vi "Unquote.vi"(1 "String":string) -> (0 "trimmed string":string)   [LabVIEW 2023, in "LV ArgParse.lvlib" / "LV Argument Parser.lvclass"]
uses:
  LV Argument Parser.lvclass
  <vilib>/Utility/error.llb/Trim Whitespace One-Sided.vi
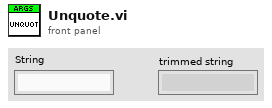
[diagram p1: front panel]
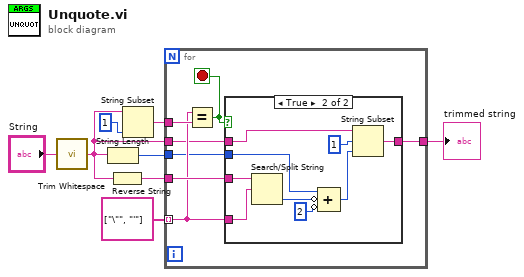
[diagram p0: block diagram]
diagram:
  n1 = call <vilib>:"Trim Whitespace.vi"("string"="String") -> ("trimmed string"=w2:string)  [unwired: 1 in]
  n2 = String Length(string=w2) -> (length=w3:i32)
  n3 = Reverse String(1:w2) -> (0:w5:string)
  n4 = String Subset(string=w2, length (rest)=1 ("length (rest)")) -> (substring=w6:string)  [unwired: 1 in]
  n5 = for {
    tunnel: w6 -> [w15]
    tunnel: w5 -> [w14]
    tunnel: string[] ["\"", "'"] -> [w13] mode=indexing
    tunnel: w3 -> [w12]
    tunnel: w2 -> [w11]
    tunnel: [w10] -> w1
    stop <- w9 stop-if-true
    n6 = Equal?(x=w13, y=w15) -> (x = y?=w9:bool)
    n7 = case shown="True" w9 {
      tunnel: w14 -> [_ w25]
      tunnel: w13 -> [_ w24]
      tunnel: w12 -> [_ w23]
      tunnel: w11 -> [w16 w21]
      tunnel: [w16 w18] -> w10
      frame False {
      }
      frame True {
        n8 = Search/Split String(string=w25, search string/char (-)=w24) -> (offset of match=w22:i32)  [unwired: 1 in, 2 out]
        n9 = Compound Arithmetic op=ADD(w23, invert w22, invert 2 ("value")) -> (w19:i32)
        n10 = String Subset(string=w21, offset (0)=1, length (rest)=w19) -> (substring=w18:string)
      }
    }
  }
  "trimmed string" <- w1
